vi "TF_postprocessing.vi"(5 "Div ch2 by:":dbl=1.0, 7 "Div ch1 by:":dbl=1.0, 9 "dt":dbl, 10 "current frequency":dbl, 11 "data":dbl[][](array[numeric]) format="%0.2f") -> (3 "ch2/ch1":cdb)   [LabVIEW 2021]
uses:
  <vilib>/Analysis/4window.llb/windowTd.ctl
  <vilib>/measure/maspectr.llb/FFT Spectrum (Mag-Phase) for 1 Chan.vi
  <vilib>/measure/NI_MAPro.lvlib
  <vilib>/Analysis/NI_AALPro.lvlib
panel:
  out "Ch1FFT Graph 2":cluster{"f0":dbl, "df":dbl, "magnitude":dbl[]}(graph)
  out "Ch2FFT Graph":cluster{"f0":dbl, "df":dbl, "magnitude":dbl[]}(graph)
  out "ch2 mag":dbl(graph)
  out "ch2 phase":dbl(graph)
  out "ch1 phase":dbl(graph)
  out "ch1 mag":dbl(graph)
  out "size(s) 2":i32
  out "size(s)":i32[](array[numeric])
  out "ch2/ch1 phase":dbl(graph)
  out "ch2/ch1 mag":dbl(graph)
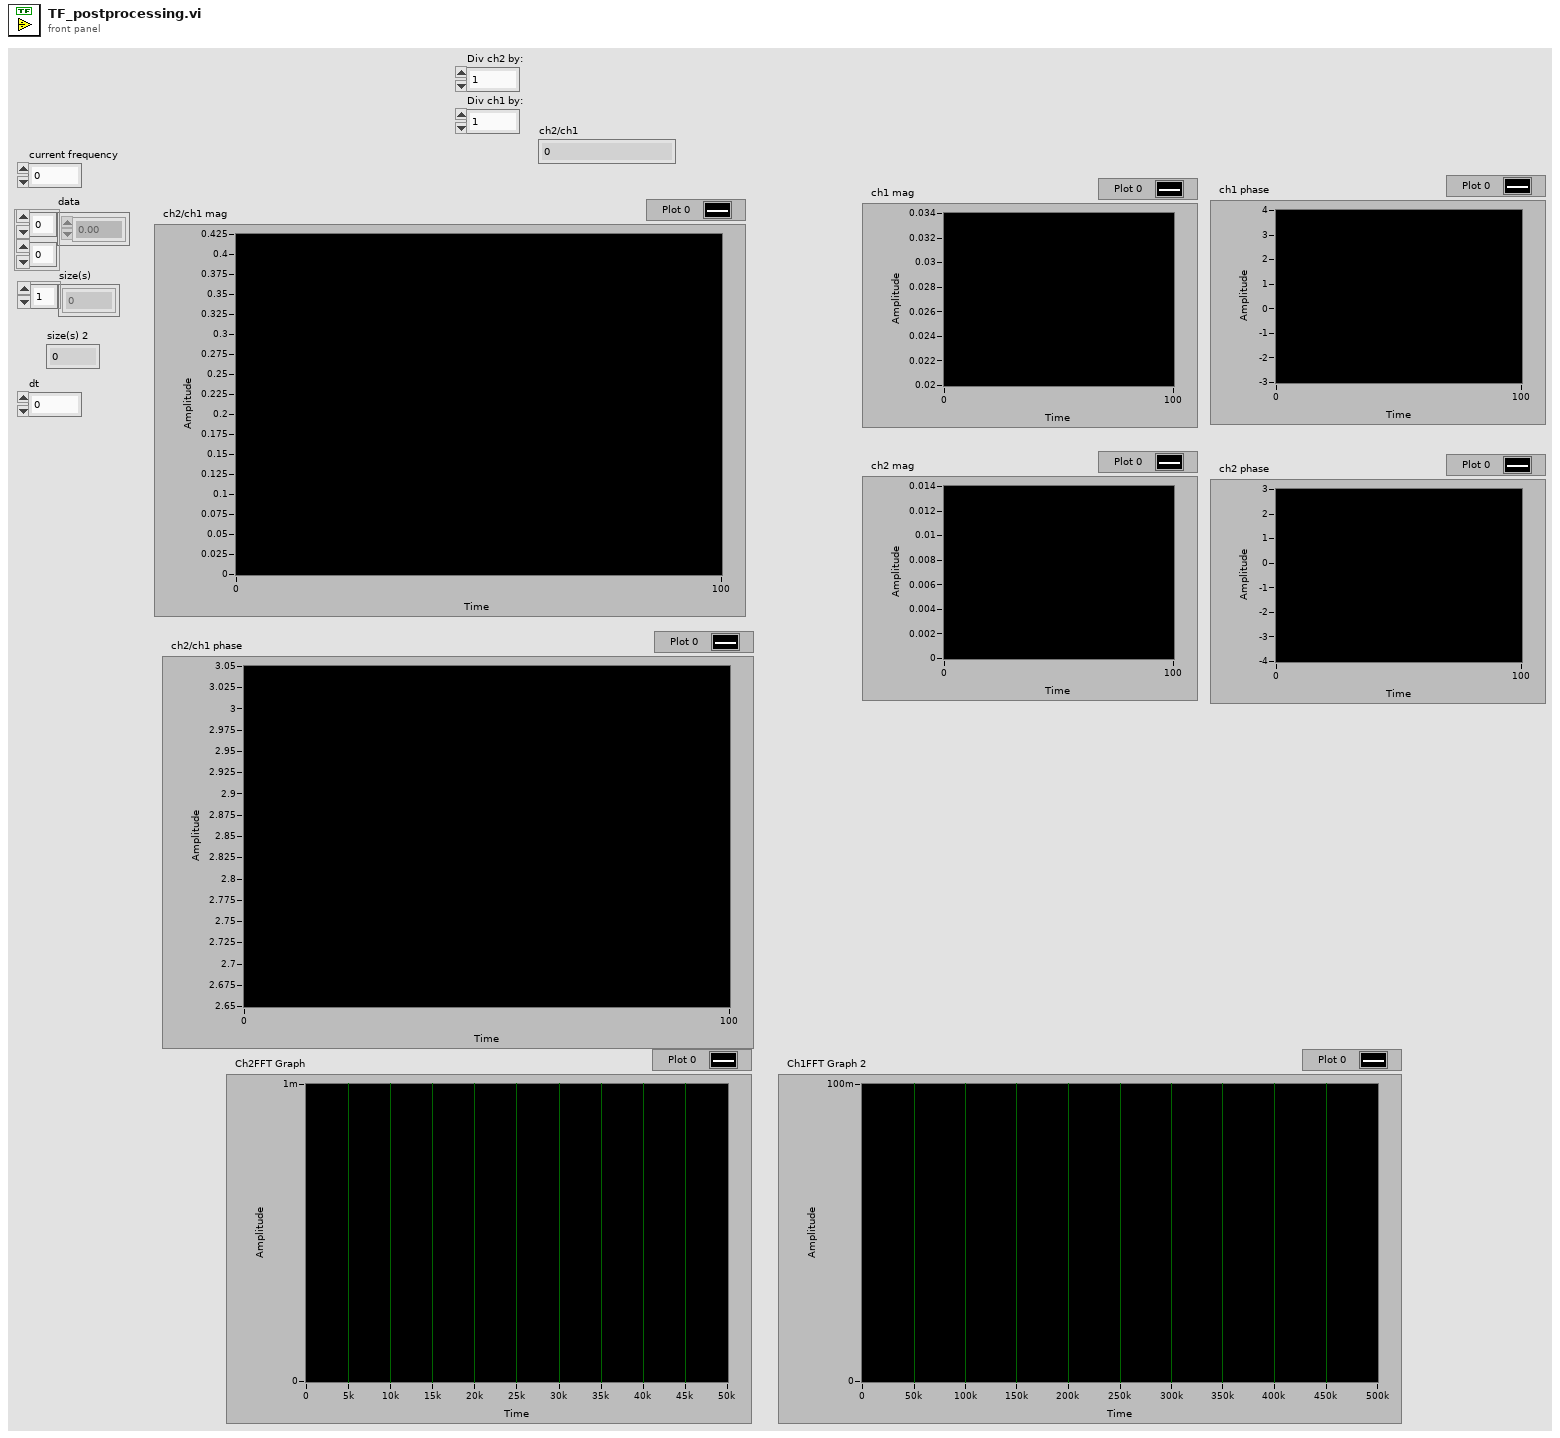
[diagram p1: front panel]
types:
  T1 = typedef "NI_AALPro.lvlib/windowTd.ctl" = u32
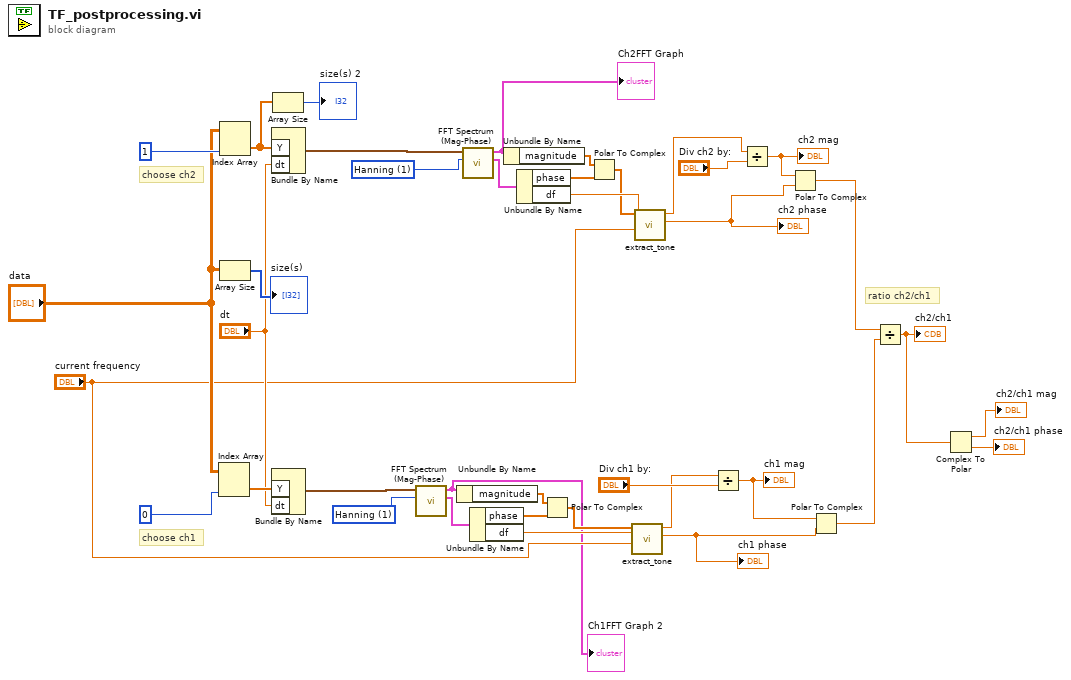
[diagram p0: block diagram]
diagram:
  w13 = T1 1 items=["Rectangle"=0, "Hanning"=1, "Hamming"=2, "Blackman-Harris"=3, "Exact Blackman"=4, "Blackman"=5, "Flat Top"=6, "4 Term B-Harris "=7, "7 Term B-Harris"=8, "Low Sidelobe"=9, "Blackman Nuttall"=11, "Triangle"=30, "Bartlett-Hanning"=31, "Bohman"=32, "Parzen"=33, "Welch"=34, "Kaiser"=60, "Dolph-Chebyshev"=61, "Gaussian"=62] ("window")
  w14 = T1 1 items=["Rectangle"=0, "Hanning"=1, "Hamming"=2, "Blackman-Harris"=3, "Exact Blackman"=4, "Blackman"=5, "Flat Top"=6, "4 Term B-Harris "=7, "7 Term B-Harris"=8, "Low Sidelobe"=9, "Blackman Nuttall"=11, "Triangle"=30, "Bartlett-Hanning"=31, "Bohman"=32, "Parzen"=33, "Welch"=34, "Kaiser"=60, "Dolph-Chebyshev"=61, "Gaussian"=62] ("window")
  # "ratio ch2/ch1"
  # "choose ch1"
  # "choose ch2"
  n1 = Index Array(array="data", index (col)=0 ("disabled index (col)")) -> (element=w29:dbl[])  [unwired: 1 in]
  n2 = Index Array(array="data", index (col)=1 ("disabled index (col)")) -> (element=w30:dbl[])  [unwired: 1 in]
  n3 = Array Size(array="data") -> (size(s)=→"size(s)":i32[])
  n4 = Bundle By Name("Y"=w30, "dt"="dt") -> (w15:waveform(dbl))  [unwired: 1 in]
  n5 = Bundle By Name("Y"=w29, "dt"="dt") -> (w12:waveform(dbl))  [unwired: 1 in]
  n6 = Array Size(array=w30) -> (size(s)=→"size(s) 2":i32)
  n7 = call-poly <vilib>:"FFT Spectrum (Mag-Phase).vi"("window"=w13, "time signal"=w12) -> ("phase"=w25:cluster{"f0":dbl, "df":dbl, "phase":dbl[]}, "magnitude"=w1:cluster{"f0":dbl, "df":dbl, "magnitude":dbl[]})  [unwired: 5 in, 3 out]
  "Ch1FFT Graph 2" <- w1
  n8 = Unbundle By Name(w1) -> ("magnitude"=w26:dbl[])
  n9 = call-poly <vilib>:"FFT Spectrum (Mag-Phase).vi"("window"=w14, "time signal"=w15) -> ("phase"=w18:cluster{"f0":dbl, "df":dbl, "phase":dbl[]}, "magnitude"=w2:cluster{"f0":dbl, "df":dbl, "magnitude":dbl[]})  [unwired: 5 in, 3 out]
  "Ch2FFT Graph" <- w2
  n10 = Unbundle By Name(w25) -> ("phase"=w24:dbl[], "df"=w22:dbl)
  n11 = Unbundle By Name(w2) -> ("magnitude"=w17:dbl[])
  n12 = Unbundle By Name(w18) -> ("phase"=w19:dbl[], "df"=w21:dbl)
  n13 = Polar To Complex(1:w24, 2:w26) -> (0:w23:cdb[])
  n14 = Polar To Complex(1:w19, 2:w17) -> (0:w20:cdb[])
  n15 = call "extract_tone.vi"("tone frequency [Hz]"="current frequency", "df"=w22, "complex fft"=w23) -> ("phase (rad)"=w9:dbl, "amplitude"=w6:dbl)  [unwired: 7 in]
  "ch1 phase" <- w9
  n16 = call "extract_tone.vi"("tone frequency [Hz]"="current frequency", "df"=w21, "complex fft"=w20) -> ("phase (rad)"=w11:dbl, "amplitude"=w4:dbl)  [unwired: 7 in]
  "ch2 phase" <- w11
  n17 = Divide(x=w6, y="Div ch1 by:") -> (x/y=w5:dbl)
  "ch1 mag" <- w5
  n18 = Divide(x=w4, y="Div ch2 by:") -> (x/y=w3:dbl)
  "ch2 mag" <- w3
  n19 = Polar To Complex(1:w11, 2:w3) -> (0:w10:cdb)
  n20 = Polar To Complex(1:w9, 2:w5) -> (0:w8:cdb)
  n21 = Divide(x=w10, y=w8) -> (x/y=w36:cdb)
  "ch2/ch1" <- w36
  n22 = Complex To Polar(r * e^(i*theta)=w36) -> (r=→"ch2/ch1 mag":dbl, theta=→"ch2/ch1 phase":dbl)
